vi "ensureVisible.vi"(4 "ymargin":i32, 6 "xmargin":i32, 8 "Error In":errorcluster, 9 "y":i32, 10 "x":i32, 11 "QScrollArea In":refnum<class "QScrollArea.lvclass">) -> (0 "Error Out":errorcluster, 3 "QScrollArea Out":refnum<class "QScrollArea.lvclass">)   [LabVIEW 2014, in "QScrollArea.lvclass"]
doc: "LabVIEW-specific documentation is not yet available. See <b>http://doc.qt.io/qt-5/QScrollArea.html#ensureVisible</b>"
uses:
  QScrollArea.lvclass
  LQ Core/LQIdentity/LQIdentity.lvclass/LQIdentity.ctl
  LQ Core/LQ Core.lvlib
  LQ Core/LQIdentity/LQIdentity.lvclass
panel:
  # "Copyright (c) 2016 Sze Howe Koh\n\nThis Source Code Form is subject to the terms of the Mozilla Public\nLicense, v. 2.0. If a copy of the MPL was not distributed with this\nfile, You can obtain one at http://mozilla.org/MPL/2.0/."
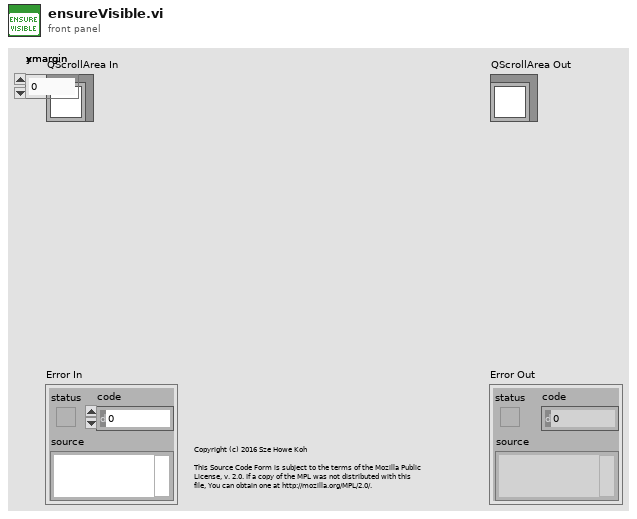
[diagram p1: front panel]
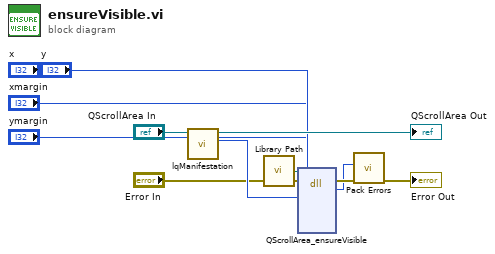
[diagram p0: block diagram]
diagram:
  n1 = call "lqManifestation.vi"("LQIdentity in"="QScrollArea In") -> ("Manifestation"=w9:u64, "LQIdentity out"=→"QScrollArea Out":refnum<class "QScrollArea.lvclass">)  [unwired: 9 in]
  n2 = call "Library Path.vi"() -> ("Library Path"=w10:path)
  n3 = dll-call lib="?" fn="QScrollArea_ensureVisible"(path in=w10, error in="Error In", "_instance"=w9, "x"="x", "y"="y", "xmargin"="xmargin", "ymargin"="ymargin") -> (error out=w7:errorcluster, w5:i32)  [unwired: 6 in, 1 out]
  n4 = call "Pack Errors.vi"("Error In"=w7, "Error Code"=w5) -> ("Error Out"=→"Error Out":errorcluster)  [unwired: 9 in]
